vi "Get Current Parameter Value - Double Float.vi"(7 "Default value":dbl format="%#_13g", 8 "error in (no error)":errorcluster, 10 "Parameter name":string, 11 "Config in":refnum<class "Config.lvclass">) -> (0 "error out":errorcluster, 2 "Value":dbl, 3 "Config out":refnum<class "Config.lvclass">)   [LabVIEW 2020, in "TALOS.lvlib" / "Classes.lvlib" / "Config.lvclass"]
doc: "Get the parameter's value (double) from the currently used configuration. Use the data type terminal to specify the output type."
uses:
  Config.lvclass
  Config.lvclass/Config.ctl
  Ancestor/Ancestor/Ancestor.lvclass/Ancestor.ctl
  FGV/Error Memory/Get Error Description.vi
  Support VIs/Get PC name.vi
  Ancestor/Ancestor/Read ID.vi
  Support VIs/Get Class Name.vi
  <vilib>/Utility/error.llb/Clear Errors.vi
  FGV/Error Memory/Error Memory Core.vi
  <vilib>/AdvancedString/Delimited String to 1D String Array.vi
  Support VIs/Circus Root Path.vi
  FGV/Error Memory/Error Crt Lvl checker.vi
  FGV/Error Memory/Error Memory Core.vi/40c8088d-b597-4017-91af-faa98e00292e.vi
  FGV/Error Memory/Error Memory Core.vi/d4a3ab98-063c-4e44-b43d-fbdcfe6c2be2.vi
  Support VIs/Global Memory.vi
  <vilib>/Utility/LVClass/Get LV Class Name.vi
  Support VIs/Is in Packed Library.vi
  Support VIs/TALOS Root path.vi
  Support VIs/Read CSV worksheet.vi
  Support VIs/Global Constants.vi
  <vilib>/Utility/error.llb/General Error Handler.vi
  Support VIs/Error Log.vi
  Ancestor/Ancestor/Ancestor.lvclass
  <vilib>/Comparison/Equal/Equal Functor/Equal Functor.lvclass
  TALOS.lvlib
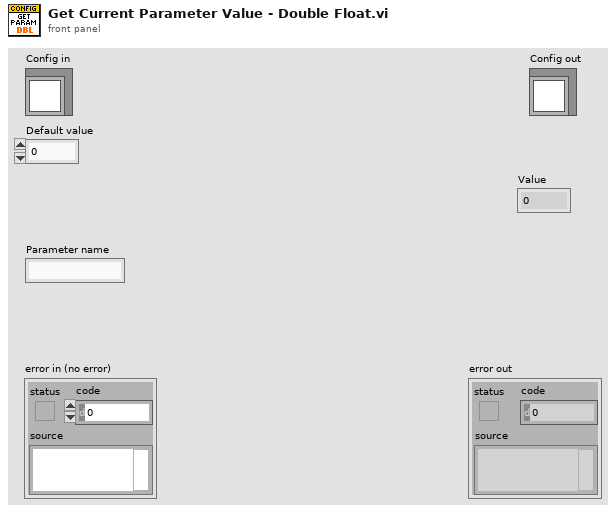
[diagram p1: front panel]
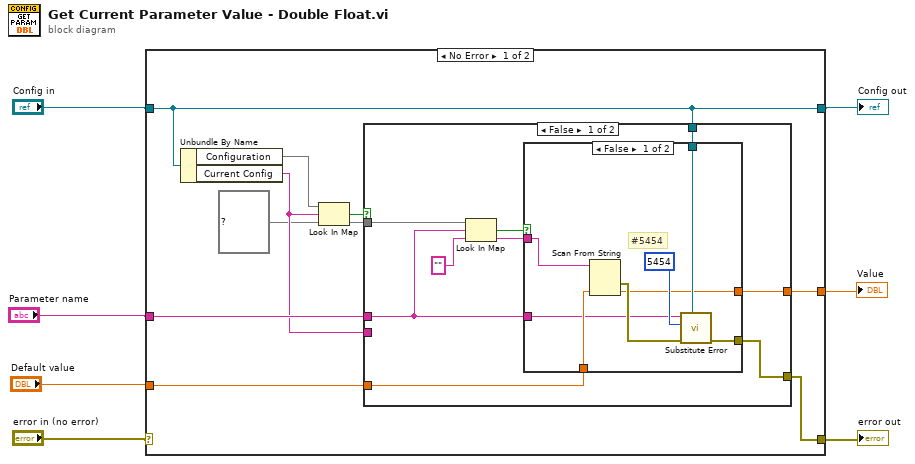
[diagram p0: block diagram]
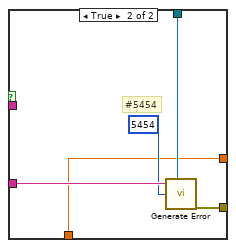
[diagram p2: hidden frame]
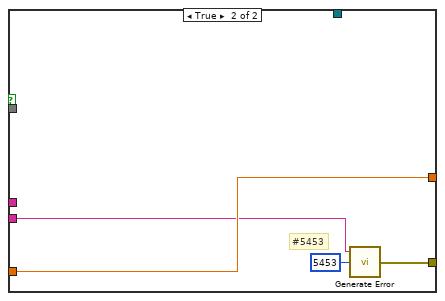
[diagram p3: hidden frame]
diagram:
  n1 = case shown="No Error" "error in (no error)" {
    selector: "error in (no error)" -> [_ w46]
    tunnel: [w14 w46] -> w1
    tunnel: [w11 w45] -> w3
    tunnel: "Config in" -> [w11 w45]
    tunnel: "Parameter name" -> [w15 _]
    tunnel: [w12 w44] -> w2
    tunnel: "Default value" -> [w10 w44]
    frame No Error {
      n2 = Unbundle By Name(w11) -> ("Configuration"=w17:map{string, map{string, string}}, "Current Config"=w9:string)
      n3 = Look In Map(map=w17, key=w9, default value=map{string, string} {}) -> (key not found?=w13:bool, value=w16:map{string, string})
      n4 = case shown="False" w13 {
        tunnel: w9 -> [_ w40]
        tunnel: w16 -> [w22 _]
        tunnel: w15 -> [w21 _]
        tunnel: [w24 w42] -> w14
        tunnel: [w26 w41] -> w12
        tunnel: w11 -> [w25 _]
        tunnel: w10 -> [w23 w41]
        frame False {
          n5 = Look In Map(map=w22, key=w21, default value="") -> (key not found?=w19:bool, value=w18:string)
          n6 = case shown="False" w19 {
            tunnel: w18 -> [w27 _]
            tunnel: [w29 w35] -> w26
            tunnel: w25 -> [w33 w38]
            tunnel: [w32 w39] -> w24
            tunnel: w21 -> [w28 w37]
            tunnel: w23 -> [w30 w35]
            frame False {
              # "#5454"
              n7 = Scan From String(input string=w27, default 1=w30) -> (error out=w34:errorcluster, output 1=w29:dbl)  [unwired: 3 in, 2 out]
              n8 = call "Substitute Error.vi"("LabVIEW Object"=w33, "error in (no error)"=w34, "Error Code"=5454, "Optional String"=w28) -> ("error out"=w32:errorcluster)  [unwired: 7 in]
            }
            frame True {
              # "#5454"
              n9 = call "Generate Error.vi"("Optional String"=w37, "Class"=w38, "Error Code"=5454) -> ("error out"=w39:errorcluster)  [unwired: 4 in]
            }
          }
        }
        frame True {
          # "#5453"
          n10 = call "Generate Error.vi"("Optional String"=w40, "Error Code"=5453) -> ("error out"=w42:errorcluster)  [unwired: 5 in]
        }
      }
    }
    frame Error {
    }
  }
  "error out" <- w1
  "Config out" <- w3
  "Value" <- w2
